vi "Render_AD_Results.vi"(4 "Background Color":u32(colorbox)=16448250, 5 "Rel._Margin":sgl=0.2, 8 "error in":errorcluster, 11 "Anomaly Detection Rresults":T1={"Image"="remote image 000001443E0F18B8", "Ground Truth"="remote image 000001443E0F3018", "Predicted Heat Map"="remote image 000001443E0F25C8", "Predicted Mask"="remote image 000001443E0F1808", "Segmentation"="remote image 000001443E0F2E08"}) -> (0 "error out":errorcluster, 3 "Anomaly Detection Results":T2(plugin-control))   [LabVIEW 2020]
uses:
  Controls/Anomaly_Detection_Results_Imgs.ctl
  <vilib>/vision/NI_Vision_Development_Module.lvlib
panel:
  out "Font Size 2":i16
  out "Font Size":i16
  in  "Desired Font (Application)":T3(ring)
  in  "[User-specified Font].Font Name":string="system font"
  in  "Horizontal Alignment":i16(ring)=1 items=["Left", "Center", "Right"]
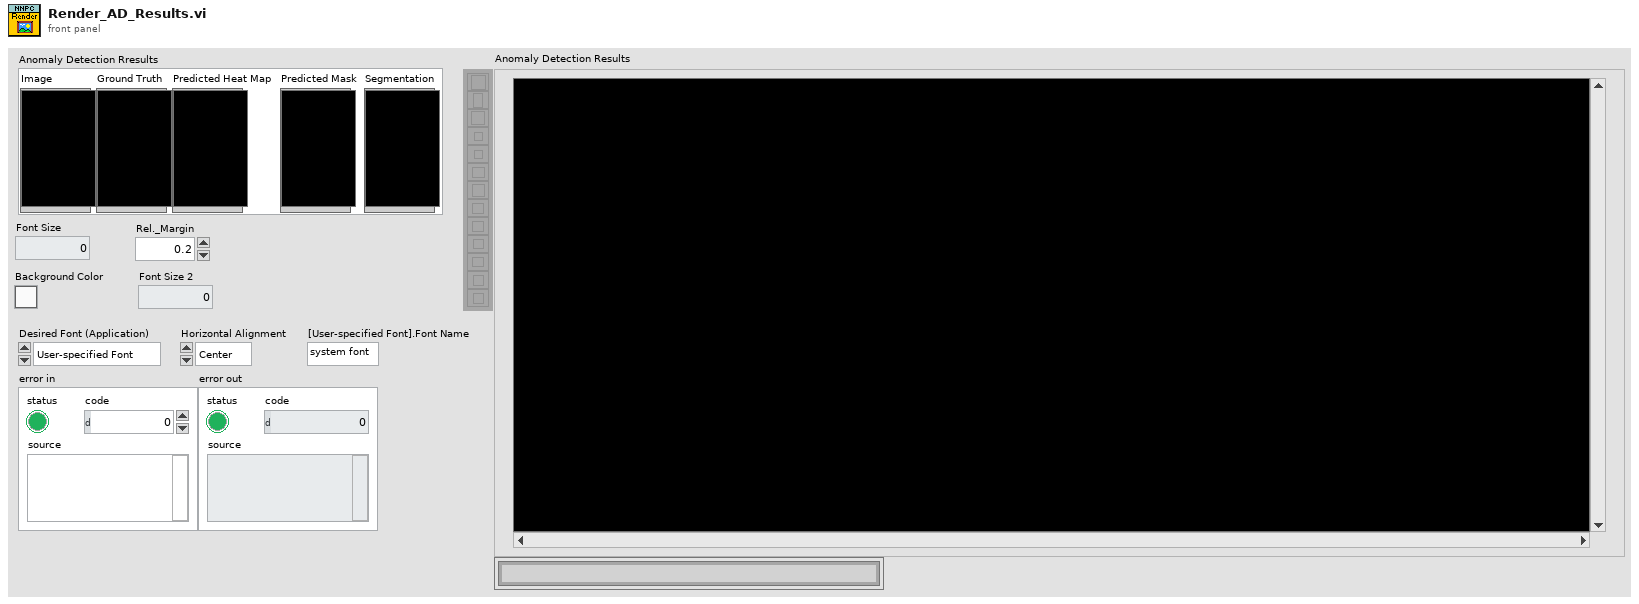
[diagram p1: front panel]
types:
  T1 = typedef "Anomaly_Detection_Results_Imgs.ctl" = cluster{"Image":T2, "Ground Truth":T2, "Predicted Heat Map":T2, "Predicted Mask":T2, "Segmentation":T2}
  T2 = typedef "IMAQ Image.ctl" = refnum<image>
  T3 = enum16{"User-specified Font", "Application Font", "System Font", "Dialog Font"}
  T4 = cluster{"Desired Font (Application)":enum16{"User-specified Font", "Application Font", "System Font", "Dialog Font"}, "[User-specified Font]":cluster{"Font Name":string, "Size":i16, "Strikeout?":bool, "Italic?":bool, "Underline?":bool, "Outline?":bool, "Shadow?":bool, "Bold?":bool, "Rotation Angle":dbl}, "Horizontal Alignment":i16, "Vertical Alignment":i16}
  T5 = typedef "Image Type" = u32
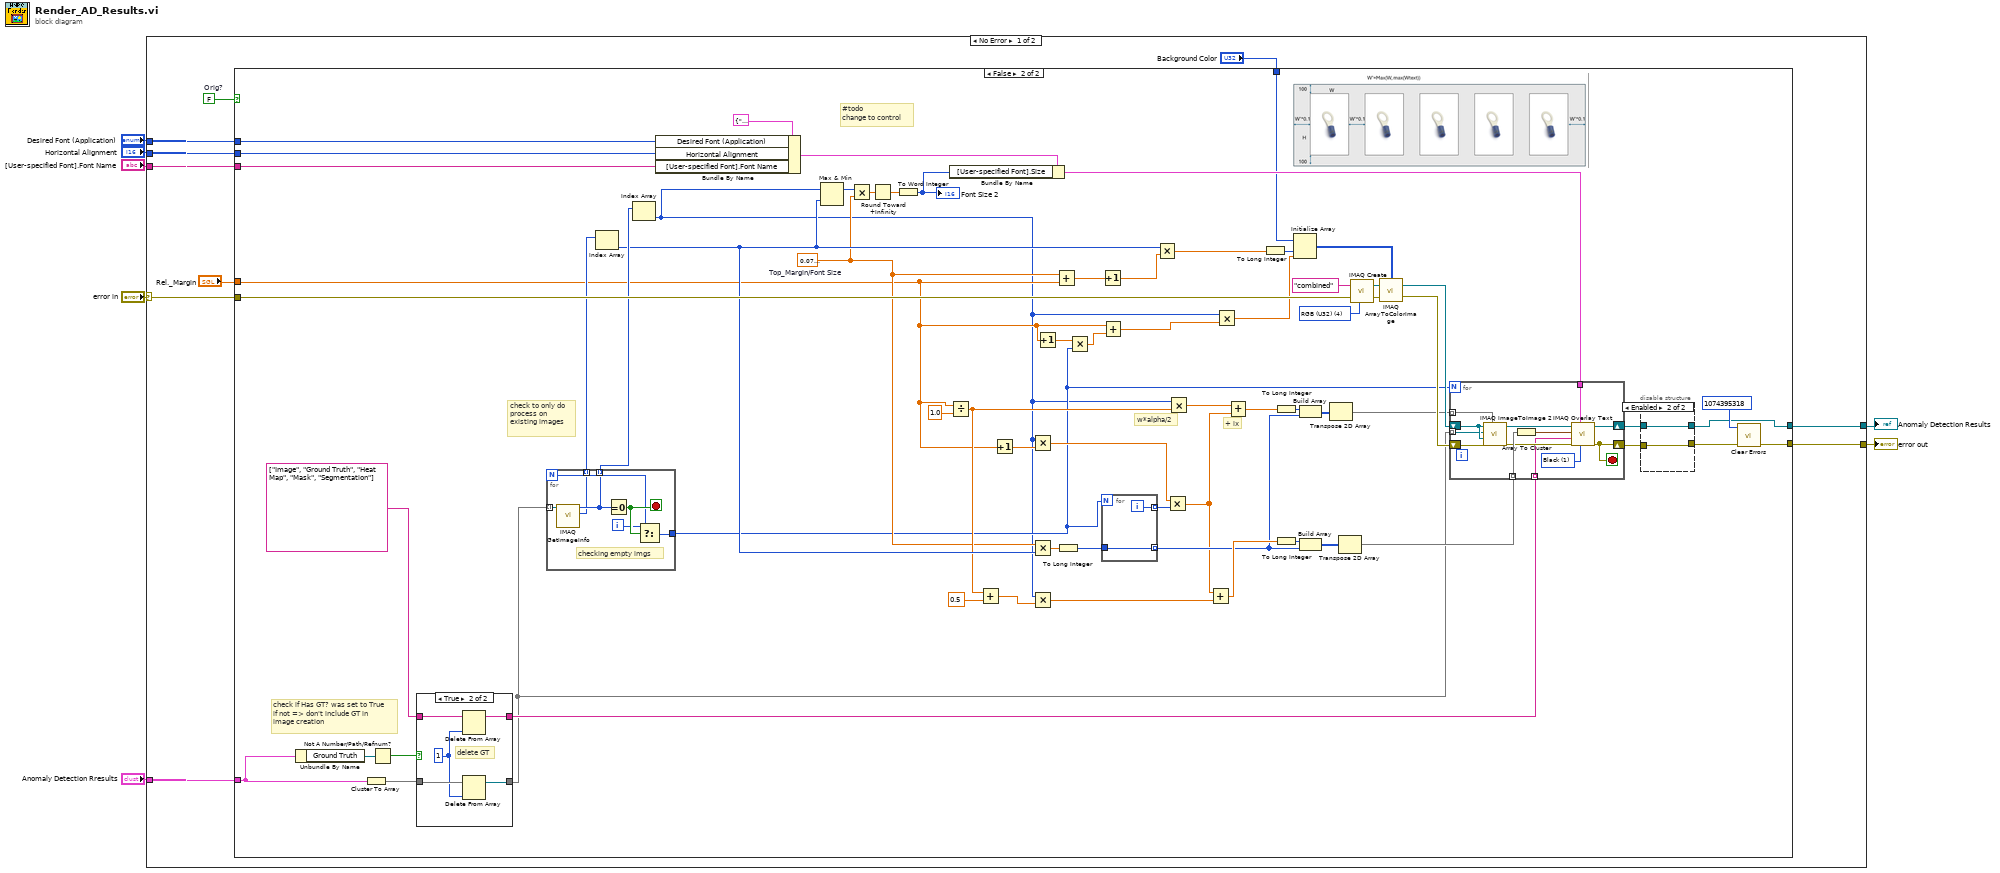
[diagram p0: block diagram]
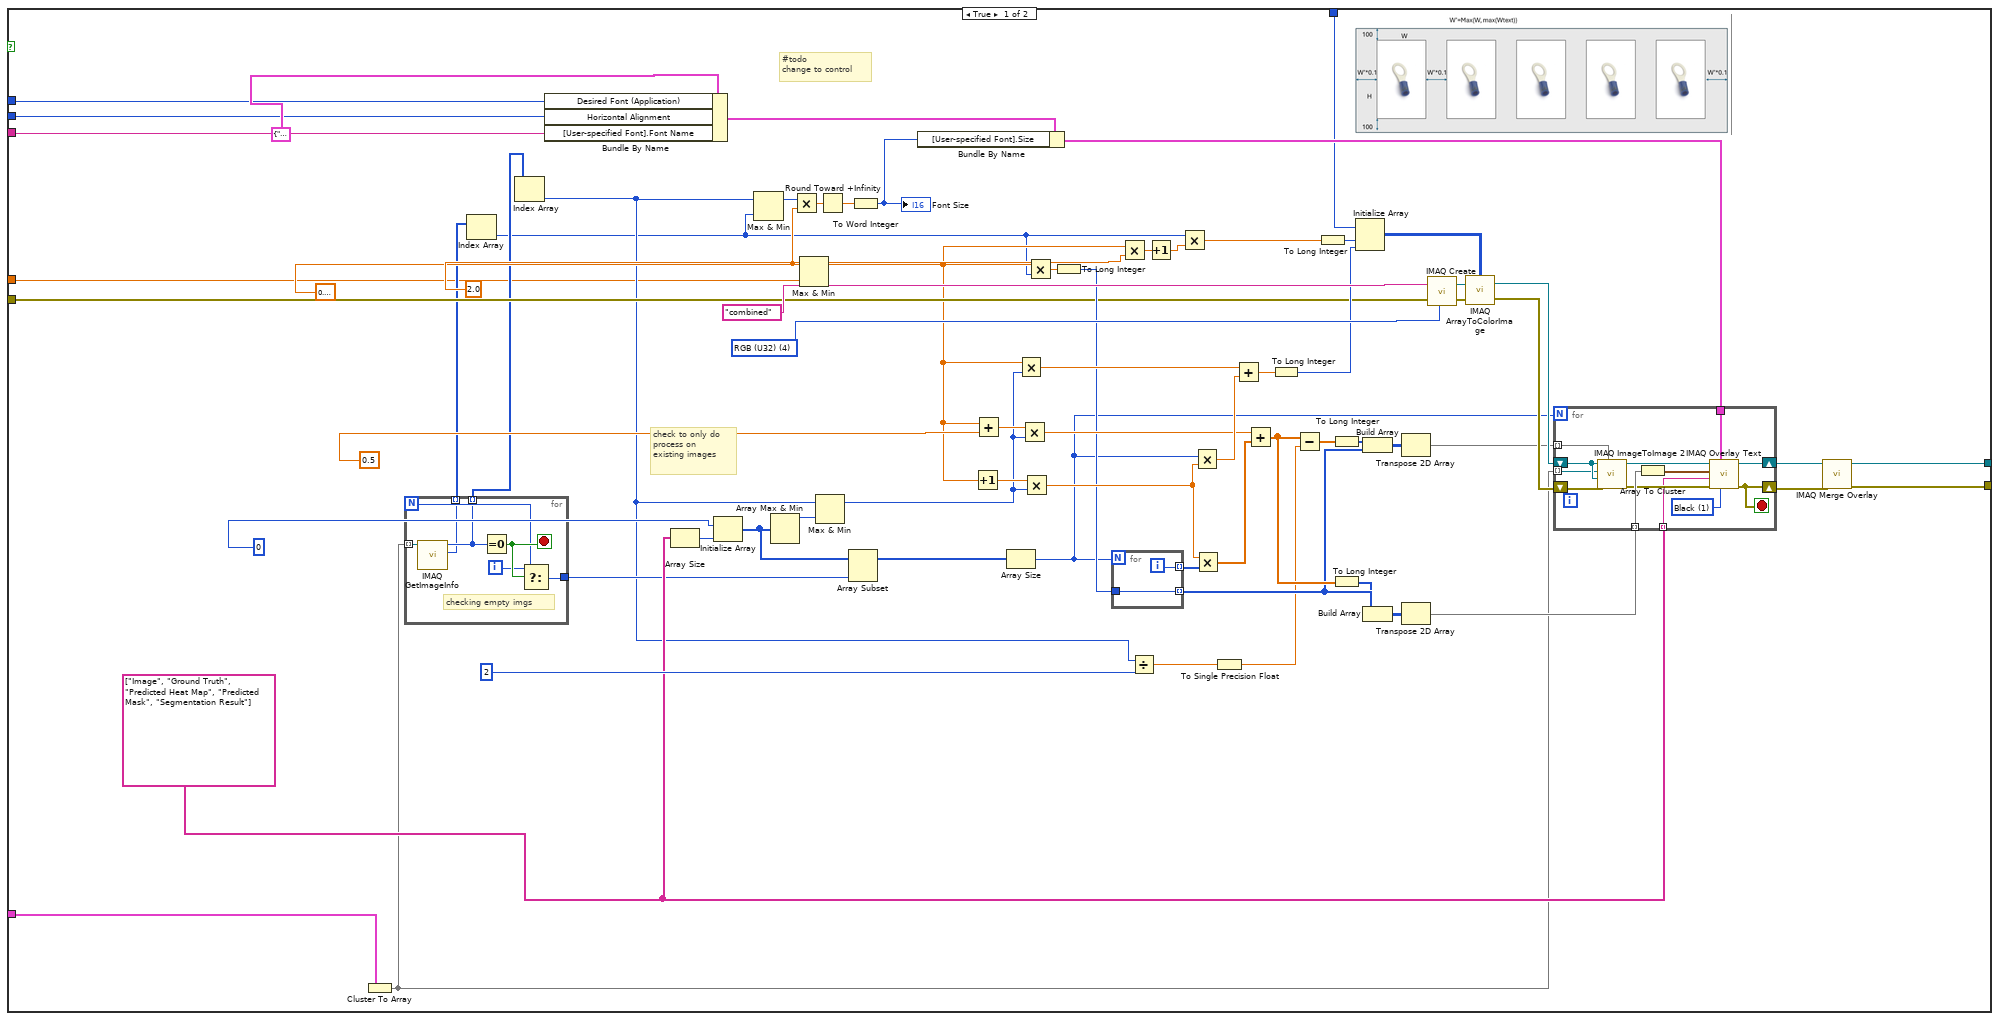
[diagram p2: hidden frame]
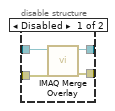
[diagram p3: hidden frame]
diagram:
  n1 = case shown="No Error" "error in" {
    selector: "error in" -> [w13 w214]
    tunnel: "Horizontal Alignment" -> [w17 _]
    tunnel: "[User-specified Font].Font Name" -> [w16 _]
    tunnel: "Desired Font (Application)" -> [w15 _]
    tunnel: [w11 w214] -> w1
    tunnel: [w12 _] -> w2
    tunnel: "Anomaly Detection Rresults" -> [w14 _]
    frame No Error {
      w10 = FALSE  # Orig?
      n2 = case shown="False" w10 {
        tunnel: w17 -> [w79 w170]
        tunnel: w16 -> [w74 w169]
        tunnel: w15 -> [w73 w168]
        tunnel: w14 -> [w43 w126]
        tunnel: w13 -> [w42 w152]
        tunnel: [w27 w111] -> w12
        tunnel: [w25 w112] -> w11
        tunnel: "Rel._Margin" -> [w19 w119]
        tunnel: "Background Color" -> [w18 w141]
        frame True {
          w33 = sgl 0.1 ("y")
          w46 = string[] ["Image", "Ground Truth", "Predicted Heat Map", "Predicted Mask", "Segmentation Result"] ("String")
          w88 = T5 4 items=["Grayscale (U8)", "Grayscale (I16)", "Grayscale (SGL)", "Complex (CSG)", "RGB (U32)", "HSL (U32)", "RGB (U64)", "Grayscale (U16)"] ("Image Type")
          # "#todo\nchange to control"
          # "check to only do process on existing images"
          n3 = Cluster To Array(cluster=w43) -> (array=w41:T2[])
          n4 = for {
            N -> [w93]
            tunnel: w41 -> [w97] mode=indexing
            tunnel: [w96] -> w28
            tunnel: [w92] -> w23 mode=indexing
            tunnel: [w91] -> w22 mode=indexing
            i -> [w94]
            stop <- w95 stop-if-true
            # "checking empty imgs"
            n5 = call "IMAQ GetImageInfo"("Image"=w97) -> ("Y Resolution"=w91:i32, "X Resolution"=w92:i32)  [unwired: 3 in, 6 out]
            n6 = Equal To 0?(x=w92) -> (x = 0?=w95:bool)
            n7 = Select(t=w94, s=w95, f=w93) -> (s? t:f=w96:i32)
          }
          n8 = Index Array(array=w22) -> (element=w20:i32)  [unwired: 1 in]
          n9 = Index Array(array=w23) -> (element=w21:i32)  [unwired: 1 in]
          n10 = Bundle By Name(cluster=T4 {"Desired Font (Application)"=enum."Application Font", "[User-specified Font]"={"Font Name"="", "Size"=12, "Strikeout?"=FALSE, "Italic?"=FALSE, "Underline?"=FALSE, "Outline?"=FALSE, "Shadow?"=FALSE, "Bold?"=FALSE, "Rotation Angle"=0.0}, "Horizontal Alignment"=0, "Vertical Alignment"=0} ("Font, Size & Style"), "Desired Font (Application)"=w73, "Horizontal Alignment"=w79, "[User-specified Font].Font Name"=w74) -> (w38:T4)
          n11 = Array Size(array=w46) -> (size(s)=w29:i32)
          n12 = Initialize Array(0 ("String width"), w29) -> (w36:i32[])
          n13 = Max & Min(x=w21, y=w20) -> (max(x,y)=w45:i32)  [unwired: 1 out]
          n14 = Array Max & Min(array=w36) -> (max value=w83:i32)  [unwired: 3 out]
          n15 = Multiply(x=w45, y=w33) -> (x*y=w44:sgl)
          n16 = Max & Min(x=w33, y=w19) -> (max(x,y)=w32:sgl)  [unwired: 1 out]
          n17 = Max & Min(x=w21, y=w83) -> (max(x,y)=w56:i32)  [unwired: 1 out]
          n18 = Round Toward +Infinity(x=w44) -> (ceil(x): smallest int >= x=w35:sgl)
          n19 = Array Subset(array=w36, length=w28) -> (w40:i32[])  [unwired: 1 in]
          n20 = To Word Integer(number=w35) -> (16bit integer=w31:i16)
          "Font Size" <- w31
          n21 = Bundle By Name(cluster=w38, "[User-specified Font].Size"=w31) -> (w37:T4)
          n22 = Increment(x=w32) -> (x+1=w61:sgl)
          n23 = Add(x=w32, y=sgl 0.5) -> (x+y=w57:sgl)
          n24 = Array Size(array=w40) -> (size(s)=w39:i32)
          n25 = Multiply(x=w32, y=w56) -> (x*y=w60:sgl)
          n26 = Multiply(x=w57, y=w56) -> (x*y=w55:sgl)
          n27 = Multiply(x=w61, y=w56) -> (x*y=w59:sgl)
          n28 = Multiply(x=w32, y=w20) -> (x*y=w34:sgl)
          n29 = To Long Integer(number=w34) -> (32bit integer=w47:i32)
          n30 = for {
            N: w39 -> [_]
            tunnel: [w90] -> w69 mode=indexing
            tunnel: [w89] -> w66 mode=indexing
            tunnel: w47 -> [w89]
            i -> [w90]
          }
          n31 = Multiply(x=w32, y=sgl 2.0) -> (x*y=w77:sgl)
          n32 = Divide(x=w21, y=2) -> (x/y=w65:dbl)
          n33 = Increment(x=w77) -> (x+1=w49:sgl)
          n34 = Multiply(x=w20, y=w49) -> (x*y=w75:sgl)
          n35 = Multiply(x=w39, y=w59) -> (x*y=w63:sgl)
          n36 = Multiply(x=w59, y=w69) -> (x*y=w68:sgl[])
          n37 = To Single Precision Float(number=w65) -> (single precision float=w50:sgl)
          n38 = Add(x=w60, y=w63) -> (x+y=w70:sgl)
          n39 = Add(x=w55, y=w68) -> (x+y=w67:sgl[])
          n40 = To Long Integer(number=w70) -> (32bit integer=w62:i32)
          n41 = Subtract(x=w67, y=w50) -> (x-y=w64:sgl[])
          n42 = To Long Integer(number=w75) -> (32bit integer=w48:i32)
          n43 = To Long Integer(number=w64) -> (32bit integer=w51:i32[])
          n44 = To Long Integer(number=w67) -> (32bit integer=w52:i32[])
          n45 = Initialize Array(w18, w48, w62) -> (w86:u32[][])
          n46 = Build Array(w51, w66) -> (w82:i32[][])
          n47 = Build Array(w52, w66) -> (w81:i32[][])
          n48 = Transpose 2D Array(2D array=w82) -> (transposed array=w54:i32[][])
          n49 = Transpose 2D Array(2D array=w81) -> (transposed array=w53:i32[][])
          n50 = call "IMAQ Create"("Image Name"="combined", "Image Type"=w88, "error in (no error)"=w42) -> ("New Image"=w85:T2, "error out"=w72:errorcluster)  [unwired: 2 in]
          n51 = call "IMAQ ArrayToColorImage"("Image Pixels (U32)"=w86, "Image"=w85, "error in (no error)"=w72) -> ("Image Out"=w84:T2, "error out"=w71:errorcluster)  [unwired: 2 in]
          n52 = for {
            N: w39 -> [_]
            tunnel: w41 -> [w108] mode=indexing
            shift-right: [w105] -> w24
            shift-left: w84 -> [w109]
            tunnel: w46 -> [w101] mode=indexing
            tunnel: w54 -> [w110] mode=indexing
            tunnel: w53 -> [w104] mode=indexing
            tunnel: w37 -> [w103]
            shift-right: [w100] -> w26
            shift-left: w71 -> [w107]
            stop <- w100 stop-if-true
            w99 = 1 items=["White", "Black", "Inverted", "Black on White", "White on Black"] ("Color")
            n53 = call "IMAQ ImageToImage 2"("Offset Left/Top"=w110, "error in (no error)"=w107, "Image Dst"=w109, "Image Src (Small)"=w108, "Image Src (Large)"=w109) -> ("error out"=w102:errorcluster, "Image Dst Out"=w106:T2)  [unwired: 5 in]
            n54 = Array To Cluster(array=w104) -> (cluster=w98:cluster{"[0]":i32, "[1]":i32})
            n55 = call "IMAQ Overlay Text"("Text Color (black)"=w99, "Font, Size & Style"=w103, "error in (no error)"=w102, "String"=w101, "Origin"=w98, "Image"=w106) -> ("error out"=w100:errorcluster, "Image Out"=w105:T2)  [unwired: 4 in]
          }
          n56 = call "IMAQ Merge Overlay"("error in (no error)"=w26, "Image Src"=w24) -> ("error out"=w25:errorcluster, "Image Dst Out"=w27:T2)  [unwired: 8 in]
        }
        frame False {
          w122 = sgl 0.08  # Top_Margin/Font Size
          w178 = T5 4 items=["Grayscale (U8)", "Grayscale (I16)", "Grayscale (SGL)", "Complex (CSG)", "RGB (U32)", "HSL (U32)", "RGB (U64)", "Grayscale (U16)"] ("Image Type")
          # "check if Has GT? was set to True\nif not => don't include GT in \nimage creation"
          # "+ ix"
          # "w*alpha/2"
          # "#todo\nchange to control"
          # "check to only do process on existing images"
          n57 = Unbundle By Name(w126) -> ("Ground Truth"=w130:T2)
          n58 = Cluster To Array(cluster=w126) -> (array=w125:T2[])
          n59 = Not A Number/Path/Refnum?(number/path/refnum=w130) -> (NaN/Path/Refnum?=w129:bool)
          n60 = case shown="True" w129 {
            tunnel: w125 -> [w207 w213]
            tunnel: [w207 w210] -> w124
            tunnel: string[] ["Image", "Ground Truth", "Heat Map", "Mask", "Segmentation"] ("String") -> [w208 w212]
            tunnel: [w208 w211] -> w127
            frame False {
            }
            frame True {
              w209 = 1 ("index")
              # "delete GT"
              n61 = Delete From Array(array=w212, index=w209) -> (array with subset deleted=w211:string[])  [unwired: 1 in, 1 out]
              n62 = Delete From Array(array=w213, index=w209) -> (array with subset deleted=w210:T2[])  [unwired: 1 in, 1 out]
            }
          }
          n63 = for {
            N -> [w189]
            tunnel: w124 -> [w193] mode=indexing
            tunnel: [w192] -> w117
            tunnel: [w188] -> w144 mode=indexing
            tunnel: [w187] -> w143 mode=indexing
            i -> [w190]
            stop <- w191 stop-if-true
            # "checking empty imgs"
            n64 = call "IMAQ GetImageInfo"("Image"=w193) -> ("Y Resolution"=w187:i32, "X Resolution"=w188:i32)  [unwired: 3 in, 6 out]
            n65 = Equal To 0?(x=w188) -> (x = 0?=w191:bool)
            n66 = Select(t=w190, s=w191, f=w189) -> (s? t:f=w192:i32)
          }
          n67 = Index Array(array=w143) -> (element=w142:i32)  [unwired: 1 in]
          n68 = Index Array(array=w144) -> (element=w115:i32)  [unwired: 1 in]
          n69 = Bundle By Name(cluster=T4 {"Desired Font (Application)"=enum."Application Font", "[User-specified Font]"={"Font Name"="", "Size"=12, "Strikeout?"=FALSE, "Italic?"=FALSE, "Underline?"=FALSE, "Outline?"=FALSE, "Shadow?"=FALSE, "Bold?"=FALSE, "Rotation Angle"=0.0}, "Horizontal Alignment"=0, "Vertical Alignment"=0} ("Font, Size & Style"), "Desired Font (Application)"=w168, "Horizontal Alignment"=w170, "[User-specified Font].Font Name"=w169) -> (w151:T4)
          n70 = Max & Min(x=w115, y=w142) -> (max(x,y)=w154:i32)  [unwired: 1 out]
          n71 = Multiply(x=w154, y=w122) -> (x*y=w153:sgl)
          n72 = Round Toward +Infinity(x=w153) -> (ceil(x): smallest int >= x=w149:sgl)
          n73 = To Word Integer(number=w149) -> (16bit integer=w147:i16)
          "Font Size 2" <- w147
          n74 = Bundle By Name(cluster=w151, "[User-specified Font].Size"=w147) -> (w150:T4)
          n75 = Divide(x=w119, y=sgl 1.0) -> (x/y=w139:sgl)
          n76 = Add(x=w139, y=sgl 0.5) -> (x+y=w160:sgl)
          n77 = Increment(x=w119) -> (x+1=w162:sgl)
          n78 = Multiply(x=w115, y=w162) -> (x*y=w134:sgl)
          n79 = Multiply(x=w122, y=w142) -> (x*y=w148:sgl)
          n80 = Multiply(x=w115, y=w160) -> (x*y=w159:sgl)
          n81 = Increment(x=w119) -> (x+1=w120:sgl)
          n82 = Add(x=w122, y=w119) -> (x+y=w123:sgl)
          n83 = To Long Integer(number=w148) -> (32bit integer=w155:i32)
          n84 = Multiply(x=w120, y=w117) -> (x*y=w118:sgl)
          n85 = Increment(x=w123) -> (x+1=w121:sgl)
          n86 = Add(x=w119, y=w118) -> (x+y=w116:sgl)
          n87 = for {
            N: w117 -> [_]
            tunnel: [w186] -> w165 mode=indexing
            tunnel: [w185] -> w163 mode=indexing
            tunnel: w155 -> [w185]
            i -> [w186]
          }
          n88 = Multiply(x=w142, y=w121) -> (x*y=w132:sgl)
          n89 = Multiply(x=w134, y=w165) -> (x*y=w138:sgl[])
          n90 = Multiply(x=w115, y=w139) -> (x*y=w135:sgl)
          n91 = Add(x=w138, y=w159) -> (x+y=w164:sgl[])
          n92 = Multiply(x=w115, y=w116) -> (x*y=w133:sgl)
          n93 = Add(x=w135, y=w138) -> (x+y=w131:sgl[])
          n94 = To Long Integer(number=w132) -> (32bit integer=w156:i32)
          n95 = To Long Integer(number=w131) -> (32bit integer=w157:i32[])
          n96 = To Long Integer(number=w164) -> (32bit integer=w158:i32[])
          n97 = Initialize Array(w141, w156, w133) -> (w176:u32[][])
          n98 = Build Array(w157, w163) -> (w173:i32[][])
          n99 = Build Array(w158, w163) -> (w172:i32[][])
          n100 = Transpose 2D Array(2D array=w173) -> (transposed array=w136:i32[][])
          n101 = Transpose 2D Array(2D array=w172) -> (transposed array=w137:i32[][])
          n102 = call "IMAQ Create"("Image Name"="combined", "Image Type"=w178, "error in (no error)"=w152) -> ("New Image"=w175:T2, "error out"=w167:errorcluster)  [unwired: 2 in]
          n103 = call "IMAQ ArrayToColorImage"("Image Pixels (U32)"=w176, "Image"=w175, "error in (no error)"=w167) -> ("Image Out"=w174:T2, "error out"=w166:errorcluster)  [unwired: 2 in]
          n104 = for {
            N: w117 -> [_]
            tunnel: w124 -> [w205] mode=indexing
            shift-right: [w202] -> w145
            shift-left: w174 -> [w206]
            tunnel: w127 -> [w198] mode=indexing
            tunnel: w137 -> [w201] mode=indexing
            tunnel: w150 -> [w200]
            shift-right: [w197] -> w146
            shift-left: w166 -> [w204]
            tunnel: w136 -> [w194] mode=indexing
            stop <- w197 stop-if-true
            w196 = 1 items=["White", "Black", "Inverted", "Black on White", "White on Black"] ("Color")
            n105 = call "IMAQ ImageToImage 2"("Offset Left/Top"=w194, "error in (no error)"=w204, "Image Dst"=w206, "Image Src (Small)"=w205, "Image Src (Large)"=w206) -> ("error out"=w199:errorcluster, "Image Dst Out"=w203:T2)  [unwired: 5 in]
            n106 = Array To Cluster(array=w201) -> (cluster=w195:cluster{"[0]":i32, "[1]":i32})
            n107 = call "IMAQ Overlay Text"("Text Color (black)"=w196, "Font, Size & Style"=w200, "error in (no error)"=w199, "String"=w198, "Origin"=w195, "Image"=w203) -> ("error out"=w197:errorcluster, "Image Out"=w202:T2)  [unwired: 4 in]
          }
          n108 = disable-structure shown="Enabled" {
            disable-tunnel: w146 -> [w182 w184]
            disable-tunnel: w145 -> [w181 w183]
            disable-tunnel: [w180 w184] -> w113
            disable-tunnel: [w179 w183] -> w111
            frame Disabled {
              n109 = call "IMAQ Merge Overlay"("error in (no error)"=w182, "Image Src"=w181) -> ("error out"=w180:errorcluster, "Image Dst Out"=w179:T2)  [unwired: 8 in]
            }
            frame Enabled {
            }
          }
          n110 = call <vilib>:"Clear Errors.vi"("error in (no error)"=w113, "specific error code to clear (0: all)"=1074395318) -> ("error out"=w112:errorcluster)  [unwired: 4 in, 1 out]
        }
      }
    }
    frame Error {
    }
  }
  "Anomaly Detection Results" <- w2
  "error out" <- w1
